vi "J1939 Message Request.vi"(0 "Destination Address":u8 format="%.0x", 5 "Source Address":u8=27, 7 "PGN":u32 format="%.0x") -> (4 "Arb ID":u32 format="%.0x", 6 "Expected Return Arb ID":u32 format="%.0x", 8 "Data":u8[](array[numeric]) format="%.0x")   [LabVIEW 2013, in "J1939.lvlib"]
uses:
  J1939.lvlib
  API Types/PGN Fields Cluster.ctl
  Frame Conversion/Convert J1939 ID to CAN Arb ID.vi
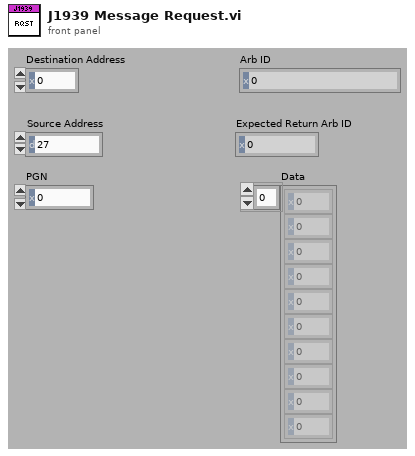
[diagram p1: front panel]
types:
  T1 = typedef "J1939.lvlib/PGN Fields Cluster.ctl" = cluster{"Reserved Bit":u8, "Data page":u8, "PDU Format":u8, "PDU Specific":u8}
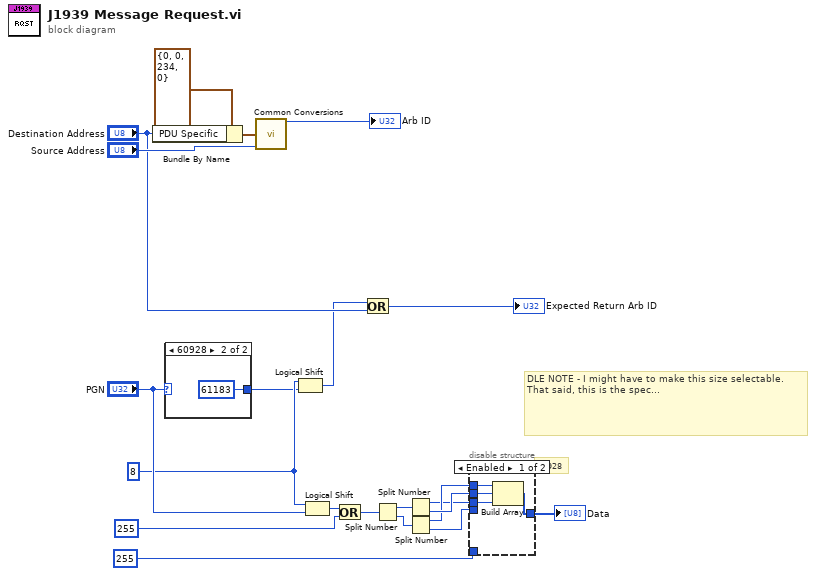
[diagram p0: block diagram]
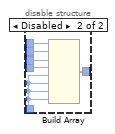
[diagram p3: hidden frame]
diagram:
  w4 = i8 8 ("y")
  # "DLE NOTE - I might have to make this size selectable.  That said, this is the spec..."
  # "60928"
  n1 = Bundle By Name(cluster=T1 {"Reserved Bit"=0, "Data page"=0, "PDU Format"=234, "PDU Specific"=0} ("PGN Fields"), "PDU Specific"="Destination Address") -> (w20:T1)
  n2 = case shown="60928" "PGN" {
    selector: "PGN" -> [w22 _]
    tunnel: [w22 u32 61183 ("PGN")] -> w3
    frame Default {
    }
    frame 60928 {
    }
  }
  n3 = call-poly "Common Conversions.vi"("PGN Fields"=w20, "Source Address"="Source Address") -> ("ID"=→"Arb ID":u32)  [unwired: 3 in, 10 out]
  n4 = Logical Shift(y=w4, x=w3) -> (x << y=w2:u32)
  n5 = Logical Shift(y=w4, x="PGN") -> (x << y=w1:u32)
  n6 = Or(x=w1, y=u32 255 ("x")) -> (x .or. y?=w15:u32)
  n7 = Or(x=w2, y="Destination Address") -> (x .or. y?=→"Expected Return Arb ID":u32)
  n8 = Split Number(x=w15) -> (hi(x)=w14:u16, lo(x)=w13:u16)
  n9 = Split Number(x=w14) -> (hi(x)=w6:u8, lo(x)=w12:u8)
  n10 = Split Number(x=w13) -> (hi(x)=w7:u8, lo(x)=w11:u8)
  n11 = disable-structure shown="Enabled" {
    disable-tunnel: w12 -> [w27 w33]
    disable-tunnel: w11 -> [_ w32]
    disable-tunnel: u8 255 ("x") -> [_ w31]
    disable-tunnel: [w26 w30] -> w8
    disable-tunnel: w7 -> [w25 w29]
    disable-tunnel: w6 -> [w24 w28]
    frame Enabled {
      n12 = Build Array(w25, w27, w24) -> (w26:u8[])
    }
    frame Disabled {
      n13 = Build Array(w29, w33, w28, w32, w31, w31, w31, w31) -> (w30:u8[])
    }
  }
  "Data" <- w8
